vi "GetDateTimeString.vi"(8 "error in (no error)":errorcluster, 11 "Generator in":refnum<class "Generator.lvclass">) -> (0 "error out":errorcluster, 3 "Generator out":refnum<class "Generator.lvclass">)   [LabVIEW 2014, in "Generator.lvlib" / "Generator.lvclass"]
uses:
  Generator.lvclass
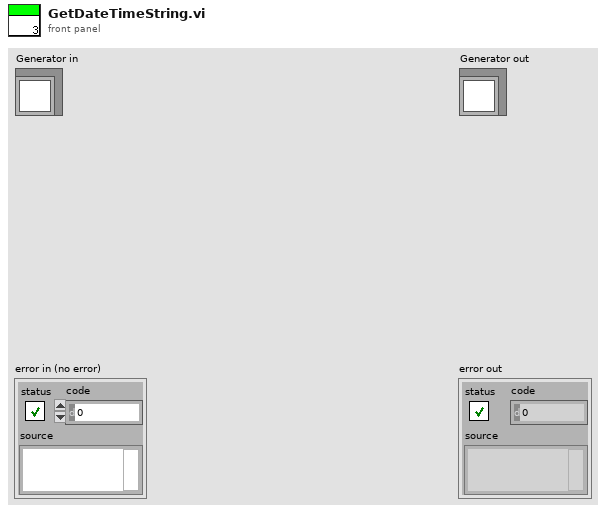
[diagram p1: front panel]
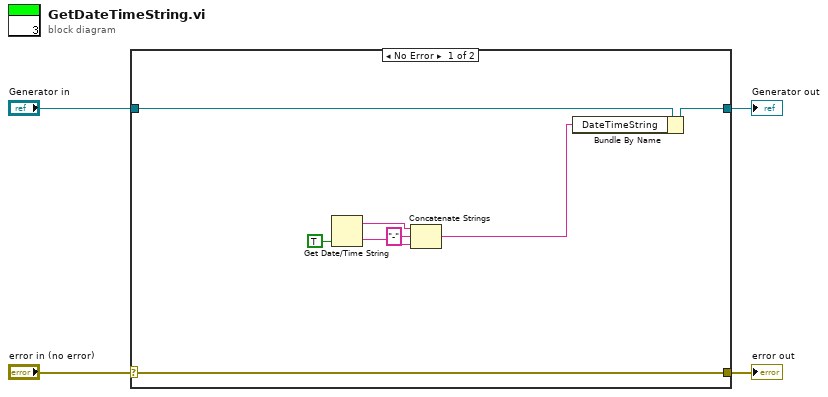
[diagram p0: block diagram]
diagram:
  n1 = case shown="No Error" "error in (no error)" {
    selector: "error in (no error)" -> [w11 w14]
    tunnel: [w11 w14] -> w3
    tunnel: [w10 w13] -> w1
    tunnel: "Generator in" -> [w12 w13]
    frame No Error {
      n2 = Get Date/Time String(want seconds? (F)=TRUE) -> (date string=w8:string, time string=w7:string)  [unwired: 2 in]
      n3 = Concatenate Strings(w8, "-" ("string"), w7) -> (w5:string)
      n4 = Bundle By Name(cluster=w12, "DateTimeString"=w5) -> (w10:refnum<class "Generator.lvclass">)
    }
    frame Error {
    }
  }
  "error out" <- w3
  "Generator out" <- w1
